vi "SetPluginNameForItemType.vi"(8 "error in (no error)":errorcluster, 9 "PluginName":string, 10 "ItemType":string, 11 "SelectedPluginStorage in":refnum<class "SelectedPluginStorage.lvclass">) -> (0 "error out":errorcluster, 3 "SelectedPluginStorage out":refnum<class "SelectedPluginStorage.lvclass">)   [LabVIEW 2014, in "SelectedPluginStorage.lvclass"]
uses:
  SelectedPluginStorage.lvclass
  SelectedPluginStorage.lvclass/SelectedPluginStorage.ctl
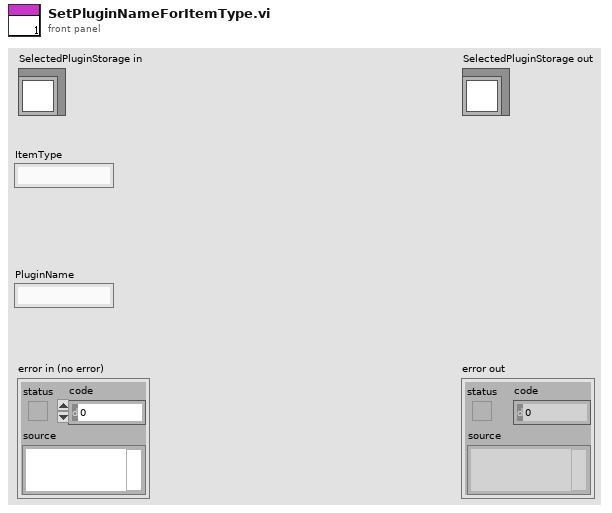
[diagram p1: front panel]
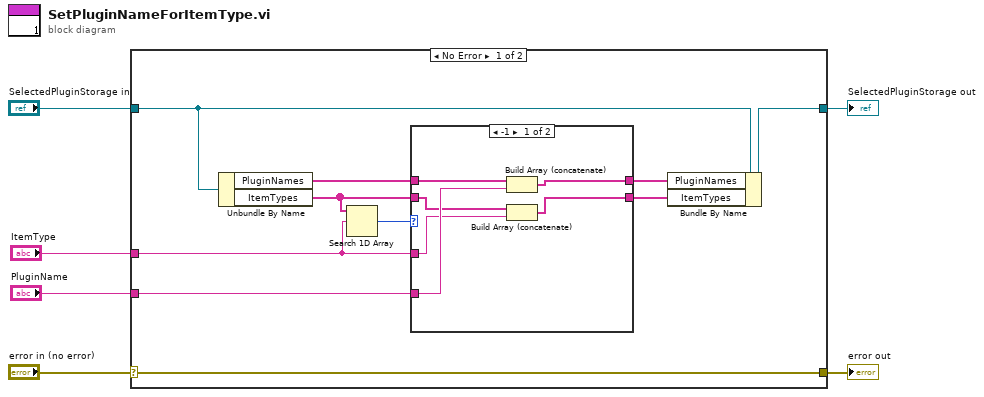
[diagram p0: block diagram]
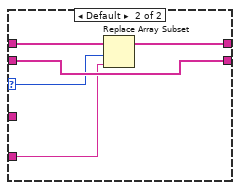
[diagram p2: hidden frame]
diagram:
  n1 = case shown="No Error" "error in (no error)" {
    selector: "error in (no error)" -> [w16 w29]
    tunnel: [w16 w29] -> w5
    tunnel: [w9 w28] -> w3
    tunnel: "SelectedPluginStorage in" -> [w15 w28]
    tunnel: "ItemType" -> [w11 _]
    tunnel: "PluginName" -> [w13 _]
    frame No Error {
      n2 = Unbundle By Name(w15) -> ("PluginNames"=w12:string[], "ItemTypes"=w10:string[])
      n3 = Search 1D Array(1D array=w10, element=w11) -> (index of element=w14:i32)  [unwired: 1 in]
      n4 = case shown="-1" w14 {
        selector: w14 -> [_ w23]
        tunnel: w13 -> [w21 w24]
        tunnel: w12 -> [w22 w27]
        tunnel: w11 -> [w19 _]
        tunnel: w10 -> [w20 w26]
        tunnel: [w18 w25] -> w8
        tunnel: [w17 w26] -> w7
        frame -1 {
          n5 = Build Array (concatenate)(w22, w21) -> (w18:string[])
          n6 = Build Array (concatenate)(w20, w19) -> (w17:string[])
        }
        frame Default {
          n7 = Replace Array Subset(array=w27, new element=w24, index=w23) -> (w25:string[])
        }
      }
      n8 = Bundle By Name(cluster=w15, "PluginNames"=w8, "ItemTypes"=w7) -> (w9:refnum<class "SelectedPluginStorage.lvclass">)
    }
    frame Error {
    }
  }
  "error out" <- w5
  "SelectedPluginStorage out" <- w3
